vi "controller_OnOff.vi"(8 "error in (no error)":errorcluster, 10 "Reference Array":cluster{"Time":dbl[], "Reference":dbl[]}, 11 "Dynamic-System in":refnum<class "Dynamic-System.lvclass">) -> (0 "error out":errorcluster, 3 "Dynamic-System out":refnum<class "Dynamic-System.lvclass">)   [LabVIEW 2025, in "Dynamic-System.lvclass"]
uses:
  Dynamic-System.lvclass
  Dynamic-System.lvclass/Dynamic-System.ctl
panel:
  out "error":dbl
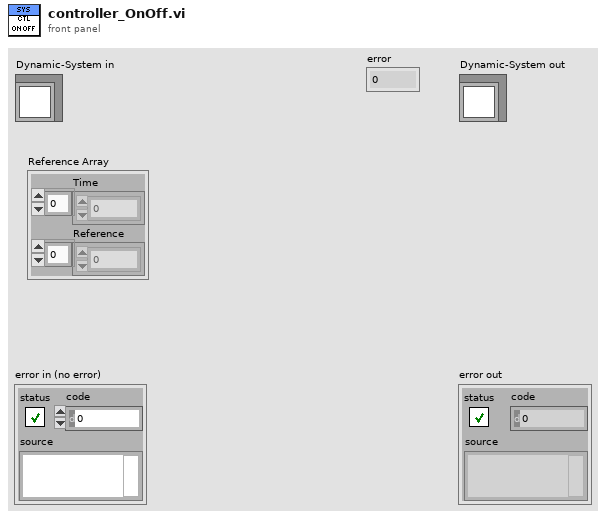
[diagram p1: front panel]
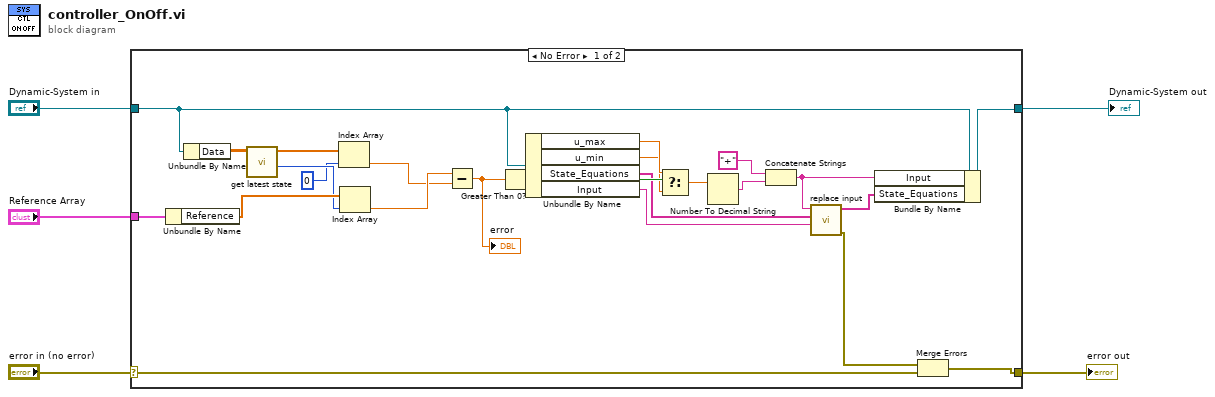
[diagram p0: block diagram]
diagram:
  n1 = case shown="No Error" "error in (no error)" {
    selector: "error in (no error)" -> [w8 w31]
    tunnel: [w6 w31] -> w4
    tunnel: [w13 w30] -> w2
    tunnel: "Dynamic-System in" -> [w16 w30]
    tunnel: "Reference Array" -> [w28 _]
    frame No Error {
      n2 = Unbundle By Name(w28) -> ("Reference"=w27:dbl[])
      n3 = Unbundle By Name(w16) -> ("Data"=w29:dbl[][])
      n4 = call "get latest state.vi"("t & X"=w29) -> ("end element"=w26:i32, "X_i"=w25:dbl[])  [unwired: 8 in, 1 out]
      n5 = Index Array(array=w25, index=0) -> (element=w22:dbl)
      n6 = Index Array(array=w27, index=w26) -> (element=w23:dbl)
      n7 = Subtract(x=w23, y=w22) -> (x-y=w21:dbl)
      "error" <- w21
      n8 = Greater Than 0?(x=w21) -> (x > 0?=w20:bool)
      n9 = Unbundle By Name(w16) -> ("u_max"=w19:dbl, "u_min"=w18:dbl, "State_Equations"=w10:string[], "Input"=w11:string)
      n10 = Select(t=w19, s=w20, f=w18) -> (s? t:f=w17:dbl)
      n11 = Number To Decimal String(number=w17) -> (decimal integer string=w15:string)  [unwired: 1 in]
      n12 = Concatenate Strings("+" ("string"), w15) -> (w12:string)
      n13 = call "replace input.vi"("Previous Input"=w11, "State_Equations in"=w10, "New Input"=w12) -> ("error out"=w7:errorcluster, "State_Equations out"=w9:string[])  [unwired: 7 in]
      n14 = Bundle By Name(cluster=w16, "Input"=w12, "State_Equations"=w9) -> (w13:refnum<class "Dynamic-System.lvclass">)
      n15 = Merge Errors(w7, w8) -> (w6:errorcluster)
    }
    frame Error {
    }
  }
  "error out" <- w4
  "Dynamic-System out" <- w2
